vi "BAM Generation Connections List_Actions.vi"(0 "Connection Cluster":T2 {"Packets"."Identifier" format="%08x"}, 1 "BAM Gen":T4, 2 "State":T1=enum."Update", 7 "index":i32, 11 "error in (no error)":errorcluster) -> (3 "BAM Gen out":T4, 4 "Connections":T2[](array[typedef]) {"Packets"."Identifier" format="%08x"}, 8 "Connection Cluster Out":T2 {"Packets"."Identifier" format="%08x"}, 15 "error out":errorcluster {"code" min=0 max=0})   [LabVIEW 2015, in "J1939 Addon Engine.lvlib"]
uses:
  J1939 Addon Engine.lvlib
  Types/BAM Generation Connections List_Ref.ctl
  Types/BAM Generation Connection Cluster.ctl
  Shared/J1939 Utilities/Types/CAN Outgoing Message Cluster.ctl
  Types/TP Connections List State.ctl
  Shared/J1939 Utilities/J1939 Utilities.lvlib
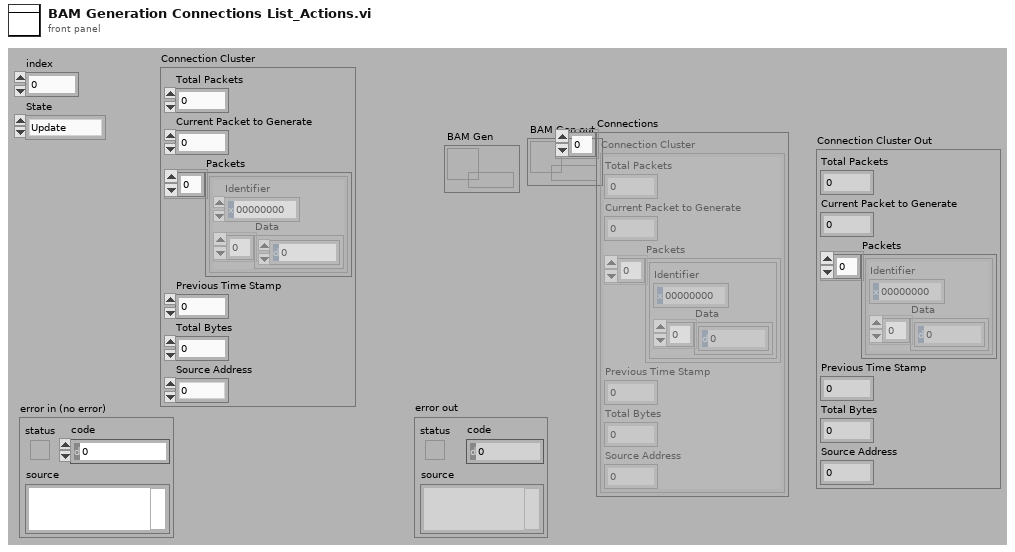
[diagram p1: front panel]
types:
  T1 = typedef "J1939 Addon Engine.lvlib/TP Connections List State.ctl" = enum16{"Add", "Update", "Get", "Remove", "Initialize"}
  T2 = typedef "J1939 Addon Engine.lvlib/BAM Generation Connection Cluster.ctl" = cluster{"Total Packets":u8, "Current Packet to Generate":u8, "Packets":T3[], "Previous Time Stamp":u32, "Total Bytes":u16, "Source Address":u8}
  T3 = typedef "J1939 Addon Shared.lvlib/J1939 Utilities.lvlib/CAN Outgoing Message Cluster.ctl" = cluster{"Identifier":u32, "Data":u8[]}
  T4 = typedef "J1939 Addon Engine.lvlib/BAM Generation Connections List_Ref.ctl" = refnum<data-value>
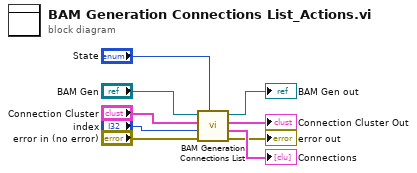
[diagram p0: block diagram]
diagram:
  n1 = call "BAM Generation Connections List.vi"("State"="State", "error in (no error)"="error in (no error)", "index"="index", "Connection Cluster"="Connection Cluster", "BAM Gen"="BAM Gen") -> ("error out"=→"error out":errorcluster, "Connections"=→"Connections":T2[], "Connection Cluster Out"=→"Connection Cluster Out":T2, "BAM Gen out"=→"BAM Gen out":T4)  [unwired: 3 in]
